vi "Mini_Test_App_box.vi"() -> ()   [LabVIEW 2015]
uses:
  Type Definitions/Mini_Test_App_Data.ctl
  <vilib>/Utility/error.llb/DialogType.ctl
panel:
  in  "UT/PASS/FAIL states":tag="Dev3/port1/line0:7"
  in  "START/STOP buttons":tag="Dev3/port0/line0:7"
  out "HP FAIL":bool
  out "HP PASS":bool
  out "HP UT":bool
  in  "Stop Hi-Pot":bool
  in  "Start Hi-Pot":bool
  out "GB FAIL":bool
  out "GB PASS":bool
  out "GB UT":bool
  in  "Stop GB":bool
  in  "Start GB":bool
  in  "Exit":bool
  # "Interface type: NI USB-6525"
  # "Warning. This app is a proof of concept and has no other purpose, \nit is not intended for production. Likewise, it has no error handling. \nUse at your own risk."
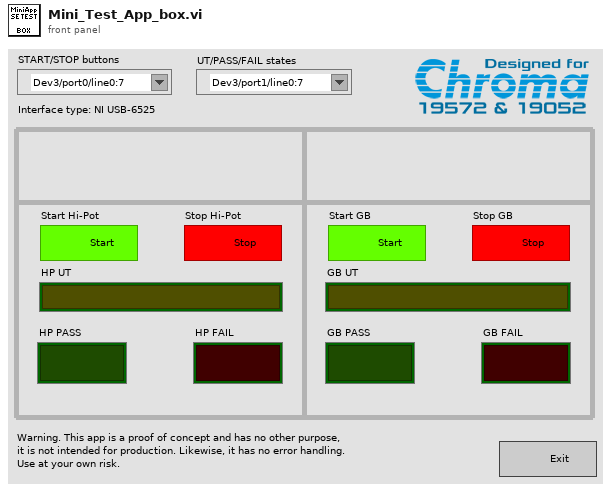
[diagram p1: front panel]
types:
  T1 = typedef "DialogType.ctl" = u16
  T2 = typedef "Mini_Test_App_Data.ctl" = cluster{"GB states":cluster{"UT":bool, "PASS":bool, "FAIL":bool}, "HP states":cluster{"UT":bool, "PASS":bool, "FAIL":bool}}
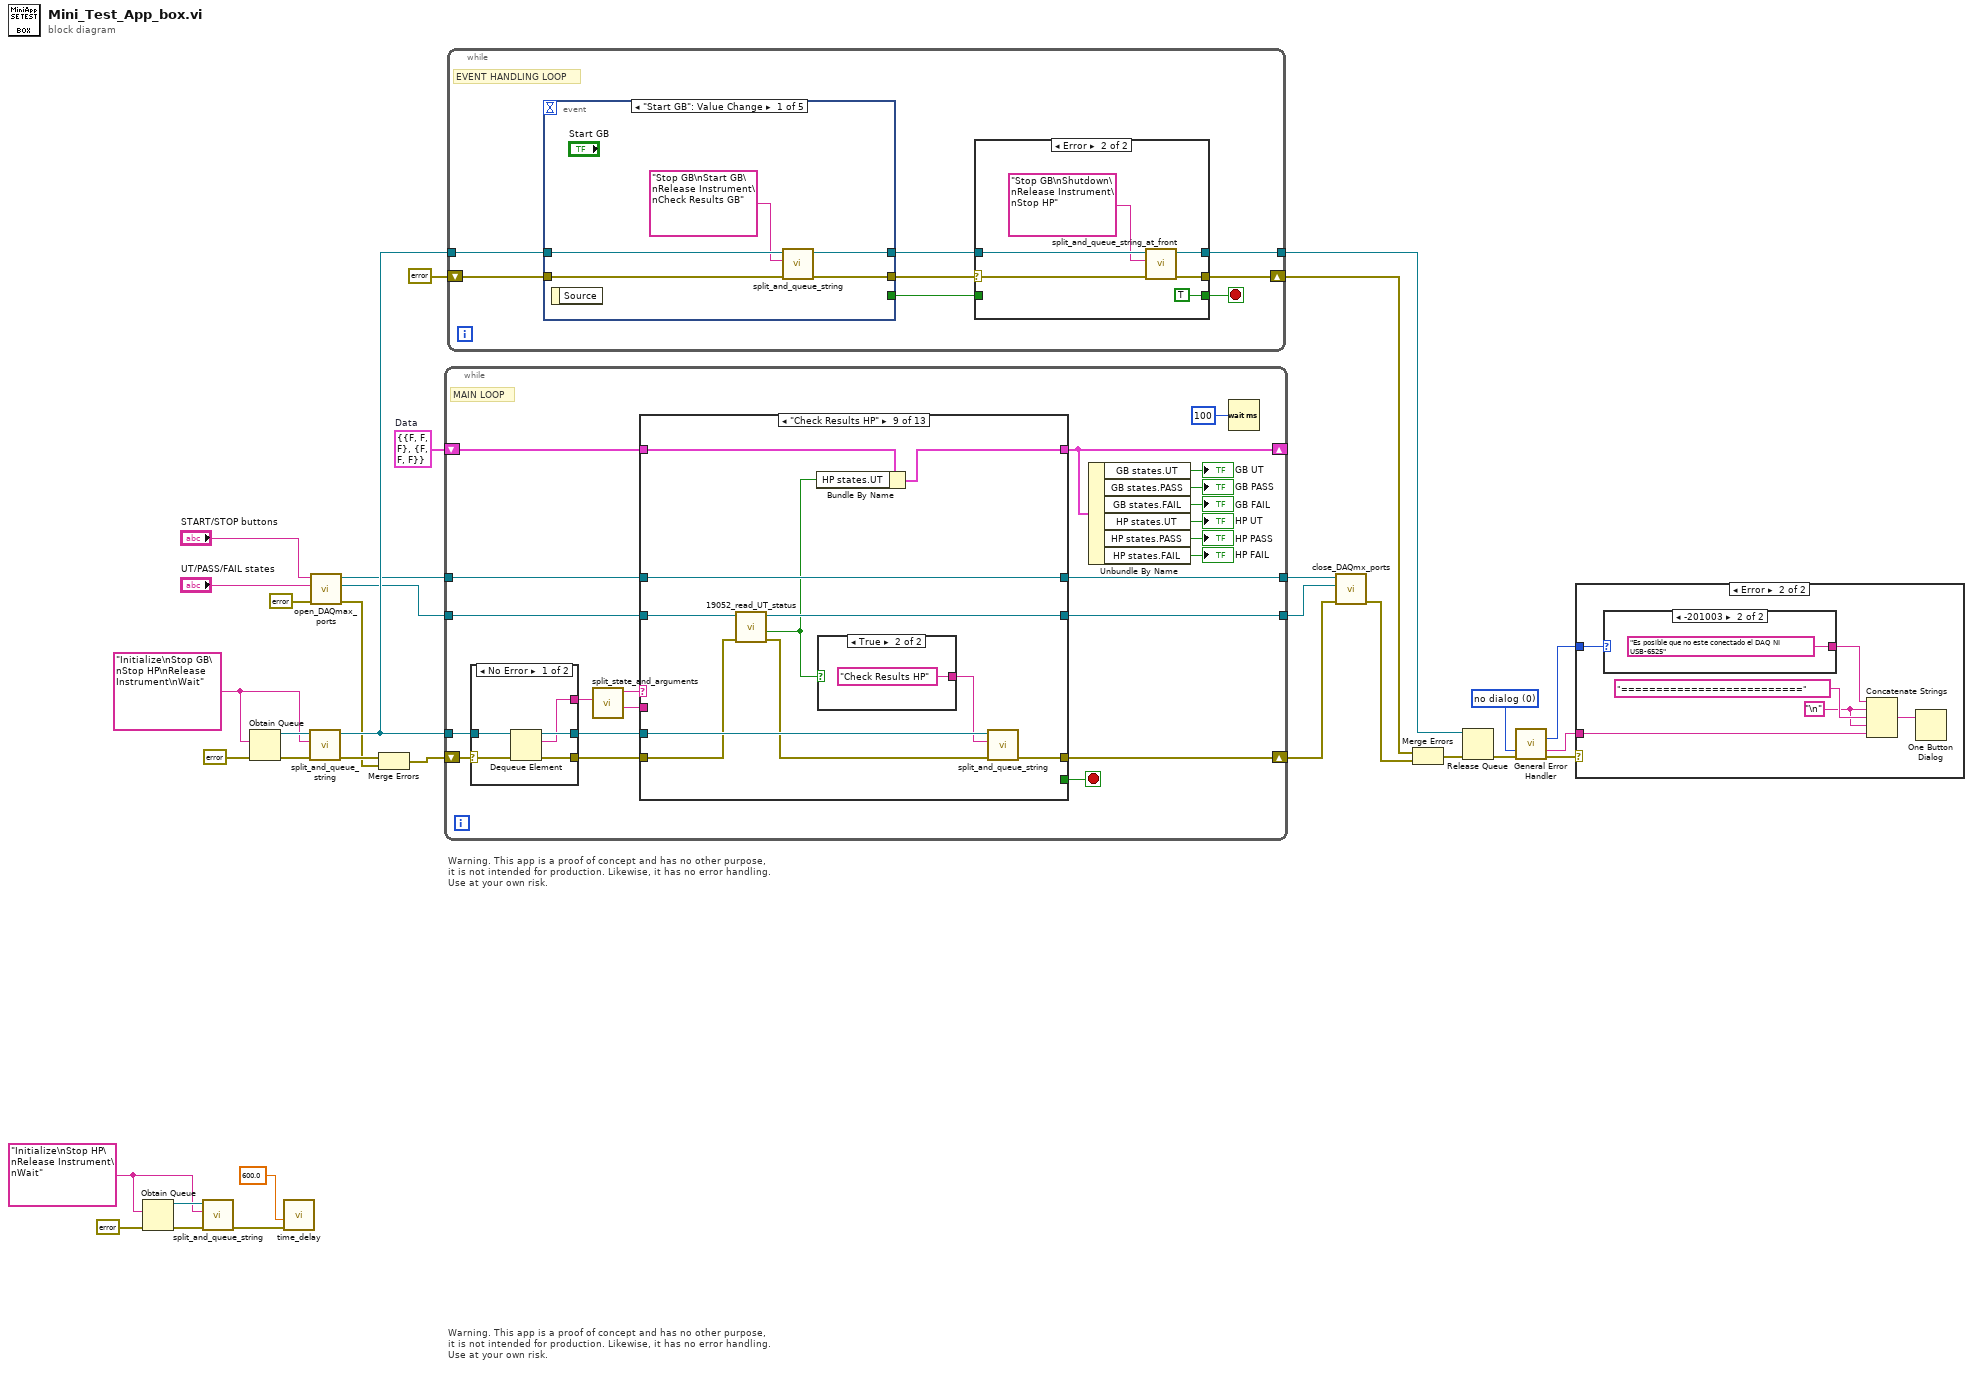
[diagram p0: block diagram]
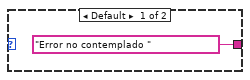
[diagram p3: hidden frame]
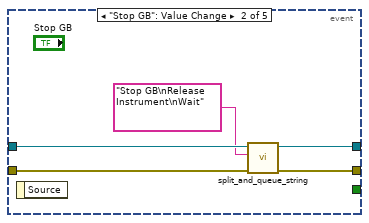
[diagram p5: hidden frame]
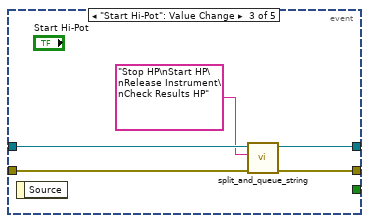
[diagram p6: hidden frame]
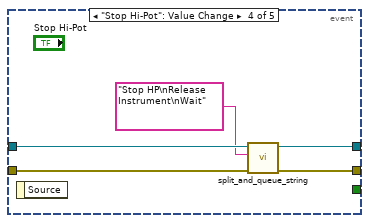
[diagram p7: hidden frame]
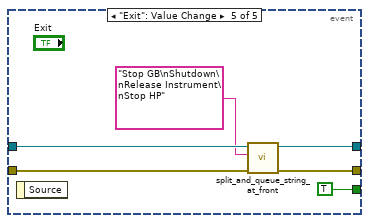
[diagram p8: hidden frame]
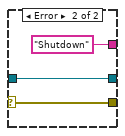
[diagram p9: hidden frame]
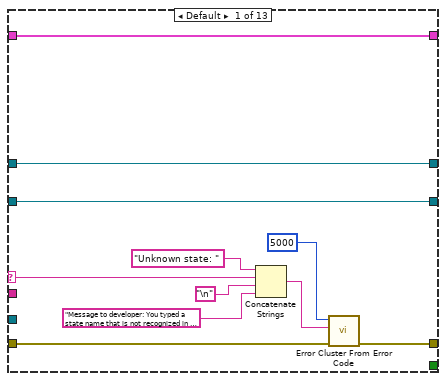
[diagram p10: hidden frame]
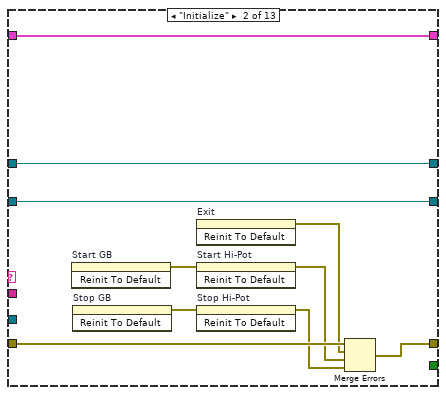
[diagram p11: hidden frame]
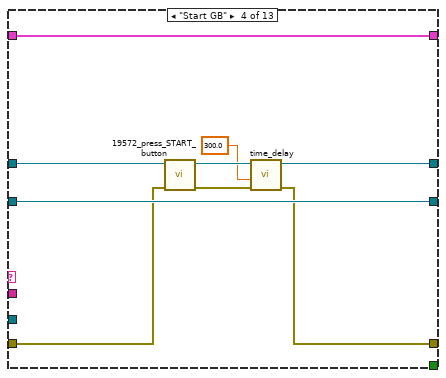
[diagram p13: hidden frame]
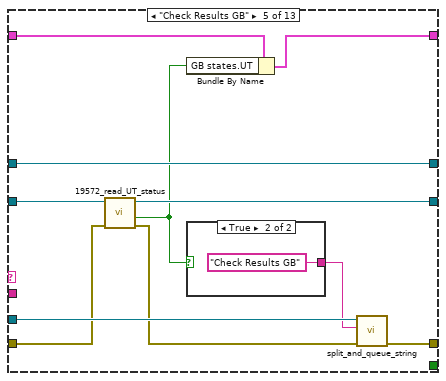
[diagram p14: hidden frame]
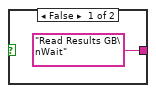
[diagram p15: hidden frame]
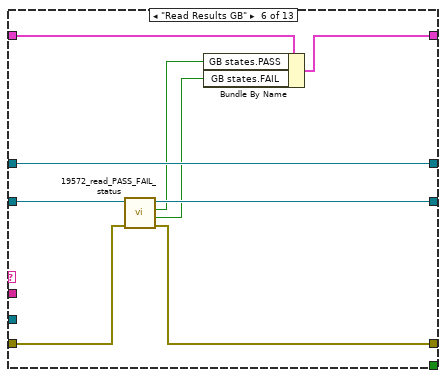
[diagram p16: hidden frame]
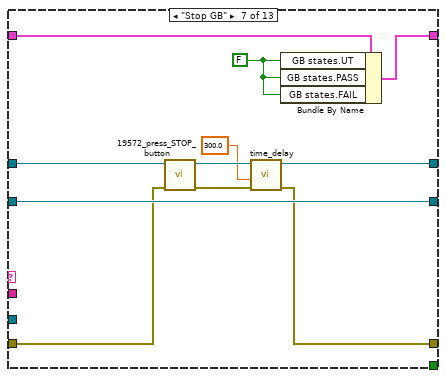
[diagram p17: hidden frame]
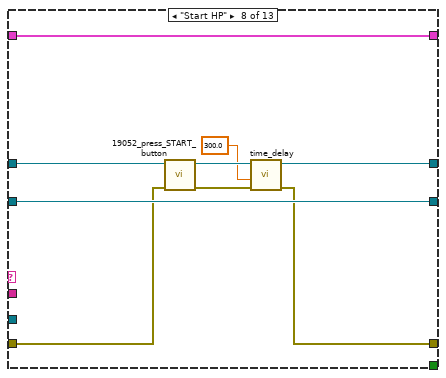
[diagram p18: hidden frame]
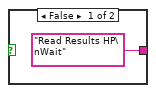
[diagram p19: hidden frame]
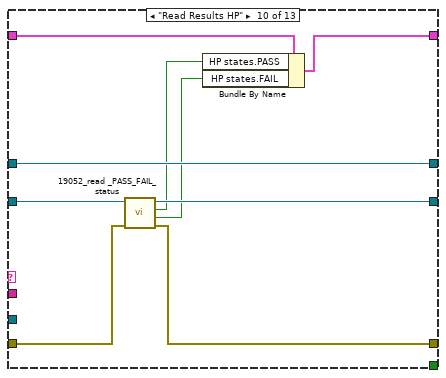
[diagram p20: hidden frame]
diagram:
  w4 = T1 0 items=["no dialog", "OK message", "continue or stop message", "OK message + warnings", "continue/stop + warnings"] ("type of dialog (OK msg:1)")
  w13 = "Initialize\nStop HP\nRelease Instrument\nWait"
  w21 = T2 {"GB states"={"UT"=FALSE, "PASS"=FALSE, "FAIL"=FALSE}, "HP states"={"UT"=FALSE, "PASS"=FALSE, "FAIL"=FALSE}}  # Data
  w23 = "Initialize\nStop GB\nStop HP\nRelease Instrument\nWait"
  # "Warning. This app is a proof of concept and has no other purpose, \nit is not intended for production. Likewise, it has no error handling. \nUse at your own risk."
  # "Warning. This app is a proof of concept and has no other purpose, \nit is not intended for production. Likewise, it has no error handling. \nUse at your own risk."
  n1 = Obtain Queue(element data type=w13, error in (no error)=errorcluster {"status"=FALSE, "code"=0, "source"=""} ("error constant")) -> (queue out=w15:refnum<queue>, error out=w14:errorcluster)  [unwired: 3 in, 1 out]
  n2 = call "split_and_queue_string.vi"("error in (no error)"=w14, "program string"=w13, "queue in"=w15) -> ("error out"=w10:errorcluster)  [unwired: 7 in, 1 out]
  n3 = Obtain Queue(element data type=w23, error in (no error)=errorcluster {"status"=FALSE, "code"=0, "source"=""} ("error constant")) -> (queue out=w27:refnum<queue>, error out=w29:errorcluster)  [unwired: 3 in, 1 out]
  n4 = call "time_delay.vi"("error in (no error)"=w10, "milliseconds to wait"=600.0) -> ()  [unwired: 9 in, 1 out]
  n5 = call "split_and_queue_string.vi"("error in (no error)"=w29, "program string"=w23, "queue in"=w27) -> ("error out"=w28:errorcluster, "queue out"=w33:refnum<queue>)  [unwired: 7 in]
  n6 = call "open_DAQmax_ports.vi"("error in (no error)"=errorcluster {"status"=FALSE, "code"=0, "source"=""} ("error constant"), "UT/PASS/FAIL states"="UT/PASS/FAIL states", "START/STOP buttons"="START/STOP buttons") -> ("error out"=w22:errorcluster, "UT/PASS/FAIL states out"=w16:refnum<k21>, "START/STOP buttons out"=w17:refnum<k21>)  [unwired: 6 in]
  n7 = Merge Errors(w28, w22) -> (w18:errorcluster)
  n8 = while {
    tunnel: w17 -> [w50]
    tunnel: w16 -> [w49]
    shift-right: [w54] -> w24
    shift-left: w18 -> [w53]
    tunnel: [w51] -> w31
    tunnel: [w48] -> w30
    tunnel: w33 -> [w46]
    shift-right: [w40] -> _
    shift-left: w21 -> [w41]
    stop <- w47 stop-if-true
    # "MAIN LOOP"
    n9 = case shown="No Error" w53 {
      selector: w53 -> [w59 w62]
      tunnel: [w58 w62] -> w52
      tunnel: w46 -> [w60 w63]
      tunnel: [w57 w63] -> w45
      tunnel: [w56 "Shutdown"] -> w42
      frame No Error {
        n10 = Dequeue Element(queue=w60, error in (no error)=w59) -> (queue out=w57:refnum<queue>, element=w56:string, error out=w58:errorcluster)  [unwired: 1 in, 1 out]
      }
      frame Error {
      }
    }
    n11 = call "split_state_and_arguments.vi"("String"=w42) -> ("Arguments"=w43:string, "State"=w44:string)  [unwired: 9 in]
    n12 = case shown="\"Check Results HP\"" w44 {
      selector: w44 -> [w66 _ _ _ _ _ _ _ _ _ _ _ _]
      tunnel: [w68 w78 w88 w90 w100 w111 w119 w129 w142 w155 w162 w169 w180] -> w54
      tunnel: w52 -> [w67 w84 w88 w93 w103 w115 w125 w130 w144 w156 w163 w170 w181]
      tunnel: [w74 w83 w87 w94 w106 w118 w126 w132 w147 w158 w168 w171 w178] -> w51
      tunnel: w50 -> [w74 w83 w87 w95 w106 w118 w127 w133 w147 w158 w164 w172 w178]
      tunnel: w49 -> [w73 w82 w86 w96 w105 w117 w128 w136 w145 w157 w167 w174 w177]
      tunnel: [w73 w82 w86 w96 w104 w116 w128 w136 w140 w154 w167 w174 w177] -> w48
      tunnel: [_ _ _ _ _ _ _ _ _ _ _ _ w179] -> w47
      tunnel: w45 -> [_ _ _ _ w107 _ _ _ w146 _ _ _ _]
      tunnel: w43 -> [_ _ _ _ _ _ _ _ _ _ _ _ _]
      tunnel: [w65 w81 w85 w89 w102 w110 w123 w135 w138 w152 w159 w173 w176] -> w40
      tunnel: w41 -> [w65 w81 w85 w89 w98 w114 w124 w135 w139 w153 w160 w173 w176]
      frame Default {
        n13 = Concatenate Strings("Unknown state: " ("string"), w66, "\n", "Message to developer: You typed a state name that is not recognized in gb test loop.") -> (w71:string)
        n14 = call <vilib>:"Error Cluster From Error Code.vi"("error in (no error)"=w67, "error message (\"\")"=w71, "error code (0)"=5000) -> ("error out"=w68:errorcluster)  [unwired: 6 in]
      }
      frame "Initialize" {
        n15 = invoke on="Start GB" class="Bool" method="Reinit To Default"() -> (error out=w80:errorcluster)  [unwired: 3 in, 2 out]
        n16 = invoke on="Stop GB" class="Bool" method="Reinit To Default"() -> (error out=w79:errorcluster)  [unwired: 3 in, 2 out]
        n17 = invoke on="Exit" class="Bool (strict)" method="Reinit To Default"() -> (error out=w75:errorcluster)  [unwired: 3 in, 2 out]
        n18 = invoke on="Start Hi-Pot" class="Bool" method="Reinit To Default"(error in=w80) -> (error out=w76:errorcluster)  [unwired: 2 in, 2 out]
        n19 = invoke on="Stop Hi-Pot" class="Bool" method="Reinit To Default"(error in=w79) -> (error out=w77:errorcluster)  [unwired: 2 in, 2 out]
        n20 = Merge Errors(w84, w75, w76, w77) -> (w78:errorcluster)
      }
      frame "Wait" {
      }
      frame "Start GB" {
        n21 = call "19572_press_START_button.vi"("error in (no error)"=w93, "task/channels in"=w95) -> ("error out"=w92:errorcluster, "task out"=w94:refnum<k21>)  [unwired: 8 in]
        n22 = call "time_delay.vi"("error in (no error)"=w92, "milliseconds to wait"=300.0) -> ("error out"=w90:errorcluster)  [unwired: 9 in]
      }
      frame "Check Results GB" {
        n23 = call "19572_read_UT_status.vi"("error in (no error)"=w103, "task/channles in"=w105) -> ("error out"=w101:errorcluster, "Under Test"=w97:bool, "task out"=w104:refnum<k21>)  [unwired: 7 in]
        n24 = Bundle By Name(cluster=w98, "GB states.UT"=w97) -> (w102:T2)
        n25 = case shown="True" w97 {
          tunnel: ["Read Results GB\nWait" "Check Results GB"] -> w99
          frame False {
          }
          frame True {
          }
        }
        n26 = call "split_and_queue_string.vi"("error in (no error)"=w101, "program string"=w99, "queue in"=w107) -> ("error out"=w100:errorcluster)  [unwired: 7 in, 1 out]
      }
      frame "Read Results GB" {
        n27 = call "19572_read_PASS_FAIL_status.vi"("error in (no error)"=w115, "task/channels in"=w117) -> ("error out"=w111:errorcluster, "Fail"=w113:bool, "Pass"=w112:bool, "task out"=w116:refnum<k21>)  [unwired: 6 in]
        n28 = Bundle By Name(cluster=w114, "GB states.PASS"=w112, "GB states.FAIL"=w113) -> (w110:T2)
      }
      frame "Stop GB" {
        w120 = FALSE
        n29 = call "19572_press_STOP_button.vi"("error in (no error)"=w125, "task/channels in"=w127) -> ("error out"=w122:errorcluster, "task out"=w126:refnum<k21>)  [unwired: 8 in]
        n30 = call "time_delay.vi"("error in (no error)"=w122, "milliseconds to wait"=300.0) -> ("error out"=w119:errorcluster)  [unwired: 9 in]
        n31 = Bundle By Name(cluster=w124, "GB states.UT"=w120, "GB states.PASS"=w120, "GB states.FAIL"=w120) -> (w123:T2)
      }
      frame "Start HP" {
        n32 = call "19052_press_START_button.vi"("error in (no error)"=w130, "task/channels in"=w133) -> ("error out"=w134:errorcluster, "task out"=w132:refnum<k21>)  [unwired: 8 in]
        n33 = call "time_delay.vi"("error in (no error)"=w134, "milliseconds to wait"=300.0) -> ("error out"=w129:errorcluster)  [unwired: 9 in]
      }
      frame "Check Results HP" {
        n34 = call "19052_read_UT_status.vi"("error in (no error)"=w144, "task/channels in"=w145) -> ("error out"=w143:errorcluster, "Under  Test"=w137:bool, "task out"=w140:refnum<k21>)  [unwired: 7 in]
        n35 = Bundle By Name(cluster=w139, "HP states.UT"=w137) -> (w138:T2)
        n36 = case shown="True" w137 {
          tunnel: ["Read Results HP\nWait" "Check Results HP"] -> w141
          frame False {
          }
          frame True {
          }
        }
        n37 = call "split_and_queue_string.vi"("error in (no error)"=w143, "program string"=w141, "queue in"=w146) -> ("error out"=w142:errorcluster)  [unwired: 7 in, 1 out]
      }
      frame "Read Results HP" {
        n38 = call "19052_read _PASS_FAIL_status.vi"("error in (no error)"=w156, "task/channels in"=w157) -> ("error out"=w155:errorcluster, "Fail"=w150:bool, "Pass"=w151:bool, "task out"=w154:refnum<k21>)  [unwired: 6 in]
        n39 = Bundle By Name(cluster=w153, "HP states.PASS"=w151, "HP states.FAIL"=w150) -> (w152:T2)
      }
      frame "Stop HP" {
        w161 = FALSE
        n40 = call "19052_press_STOP_button.vi"("error in (no error)"=w163, "task/channels in"=w164) -> ("error out"=w165:errorcluster, "task out"=w168:refnum<k21>)  [unwired: 8 in]
        n41 = call "time_delay.vi"("error in (no error)"=w165, "milliseconds to wait"=300.0) -> ("error out"=w162:errorcluster)  [unwired: 9 in]
        n42 = Bundle By Name(cluster=w160, "HP states.UT"=w161, "HP states.PASS"=w161, "HP states.FAIL"=w161) -> (w159:T2)
      }
      frame "Release Instrument" {
        n43 = call "19XX2_release_ALL.vi"("error in (no error)"=w170, "Refnum in"=w172) -> ("error out"=w169:errorcluster, "Refnum out"=w171:refnum<k21>)  [unwired: 8 in]
      }
      frame "Shutdown" {
        w179 = TRUE
        n44 = property on="Exit" class="Bool (strict)"("Val(Sgnl)"=w179) -> (error out=w175:errorcluster)  [unwired: 2 in, 1 out]
        n45 = Merge Errors(w181, w175) -> (w180:errorcluster)
      }
    }
    n46 = Unbundle By Name(w40) -> ("GB states.UT"=→"GB UT":bool, "GB states.PASS"=→"GB PASS":bool, "GB states.FAIL"=→"GB FAIL":bool, "HP states.UT"=→"HP UT":bool, "HP states.PASS"=→"HP PASS":bool, "HP states.FAIL"=→"HP FAIL":bool)
    n47 = Wait (ms)(milliseconds to wait=u32 100) -> ()  [unwired: 1 out]
  }
  n48 = while {
    shift-right: [w184] -> w19
    shift-left: errorcluster {"status"=FALSE, "code"=0, "source"=""} ("error constant") -> [w189]
    tunnel: w33 -> [w188]
    tunnel: [w186] -> w26
    stop <- w182 stop-if-true
    # "EVENT HANDLING LOOP"
    n49 = event shown="[0] \"Start GB\": Value Change" {
      selector: _ -> [_ _ _ _ _]
      dyn-events: _ -> [_ _ _ _ _]
      timeout: _ -> [_ _ _ _ _]
      tunnel: [w203 w207 w212 w217 w219] -> w185
      tunnel: w189 -> [w199 w208 w213 w218 w224]
      tunnel: w188 -> [w202 w206 w211 w216 w223]
      tunnel: [w201 w205 w210 w215 w222] -> w187
      tunnel: [_ _ _ _ TRUE] -> w183
      event "Start GB": Value Change {
        n50 = event-data() -> ()  [unwired: 1 in, 1 out]
        n51 = call "split_and_queue_string.vi"("error in (no error)"=w199, "program string"="Stop GB\nStart GB\nRelease Instrument\nCheck Results GB", "queue in"=w202) -> ("error out"=w203:errorcluster, "queue out"=w201:refnum<queue>)  [unwired: 7 in]
      }
      event "Stop GB": Value Change {
        n52 = event-data() -> ()  [unwired: 1 in, 1 out]
        n53 = call "split_and_queue_string.vi"("error in (no error)"=w208, "program string"="Stop GB\nRelease Instrument\nWait", "queue in"=w206) -> ("error out"=w207:errorcluster, "queue out"=w205:refnum<queue>)  [unwired: 7 in]
      }
      event "Start Hi-Pot": Value Change {
        n54 = event-data() -> ()  [unwired: 1 in, 1 out]
        n55 = call "split_and_queue_string.vi"("error in (no error)"=w213, "program string"="Stop HP\nStart HP\nRelease Instrument\nCheck Results HP", "queue in"=w211) -> ("error out"=w212:errorcluster, "queue out"=w210:refnum<queue>)  [unwired: 7 in]
      }
      event "Stop Hi-Pot": Value Change {
        n56 = event-data() -> ()  [unwired: 1 in, 1 out]
        n57 = call "split_and_queue_string.vi"("error in (no error)"=w218, "program string"="Stop HP\nRelease Instrument\nWait", "queue in"=w216) -> ("error out"=w217:errorcluster, "queue out"=w215:refnum<queue>)  [unwired: 7 in]
      }
      event "Exit": Value Change {
        n58 = event-data() -> ()  [unwired: 1 in, 1 out]
        n59 = call "split_and_queue_string_at_front.vi"("error in (no error)"=w224, "program string"="Stop GB\nShutdown\nRelease Instrument\nStop HP", "queue in"=w223) -> ("error out"=w219:errorcluster, "queue out"=w222:refnum<queue>)  [unwired: 7 in]
      }
    }
    n60 = case shown="Error" w185 {
      selector: w185 -> [w191 w196]
      tunnel: w187 -> [w192 w198]
      tunnel: [w192 w197] -> w186
      tunnel: [w191 w194] -> w184
      tunnel: w183 -> [w190 _]
      tunnel: [w190 TRUE] -> w182
      frame No Error {
      }
      frame Error {
        n61 = call "split_and_queue_string_at_front.vi"("error in (no error)"=w196, "program string"="Stop GB\nShutdown\nRelease Instrument\nStop HP", "queue in"=w198) -> ("error out"=w194:errorcluster, "queue out"=w197:refnum<queue>)  [unwired: 7 in]
      }
    }
  }
  n62 = call "close_DAQmx_ports.vi"("error in (no error)"=w24, "task/channels in 2"=w30, "task/channels in 1"=w31) -> ("error out"=w25:errorcluster)  [unwired: 8 in]
  n63 = Merge Errors(w19, w25) -> (w20:errorcluster)
  n64 = Release Queue(queue=w26, error in (no error)=w20) -> (error out=w11:errorcluster)  [unwired: 1 in, 2 out]
  n65 = call <vilib>:"General Error Handler.vi"("type of dialog (OK msg:1)"=w4, "error in (no error)"=w11) -> ("code out"=w5:i32, "message"=w6:string, "error out"=w7:errorcluster)  [unwired: 9 in, 2 out]
  n66 = case shown="Error" w7 {
    tunnel: w5 -> [_ w230]
    tunnel: w6 -> [_ w228]
    frame No Error {
    }
    frame Error {
      w225 = "\n"
      n67 = case shown="-201003" w230 {
        tunnel: ["Error no contemplado " "Es posible que no este conectado el DAQ NI USB-6525"] -> w229
        frame Default {
        }
        frame -201003 {
        }
      }
      n68 = Concatenate Strings(w229, w225, "==========================", w225, w228) -> (w227:string)
      n69 = One Button Dialog(message=w227) -> ()  [unwired: 1 in, 1 out]
    }
  }
